vi "abre_help_adq.vi"(1 "nome":string) -> (0 "Erro":bool)   [LabVIEW 2019]
doc: "Este vi abre arquivos pelo Acrobat (.pdf).\nNome PDF - nome do arquivo que deseja abrir. Ele deve estar na subpasta data do mesmo diretório que este vi.\nOk - se false é pq ocorreu algum erro ao procurar o arquivo. Para saber qual erro ocorreu, veja em error out. Caso contrário, o arquivo é aberto."
panel:
  out "appended path":path
  out "error out":errorcluster
  in  "error in (no error)":errorcluster
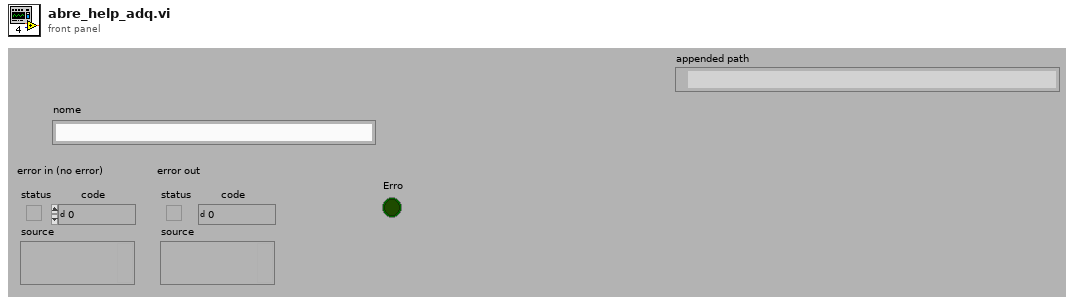
[diagram p1: front panel]
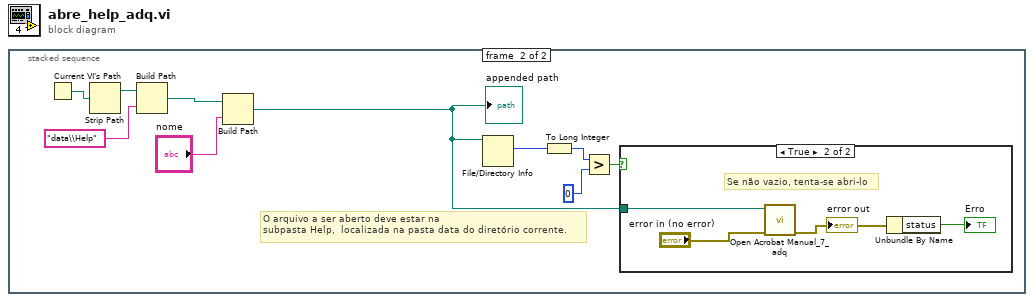
[diagram p0: block diagram]
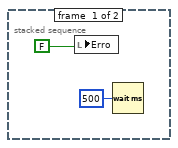
[diagram p2: hidden frame]
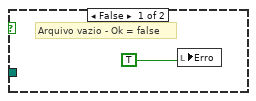
[diagram p3: hidden frame]
diagram:
  n1 = stacked-sequence {
    frame #0 {
      n2 = local write "Erro"(FALSE) -> ()
      n3 = Wait (ms)(milliseconds to wait=u32 500) -> ()  [unwired: 1 out]
    }
    frame #1 {
      # "O arquivo a ser aberto deve estar na \nsubpasta Help,  localizada na pasta data do diretório corrente."
      n4 = Current VI's Path() -> (path=w7:path)
      n5 = Strip Path(path=w7) -> (stripped path=w6:path)  [unwired: 1 out]
      n6 = Build Path(base path=w6, name or relative path="data\\Help") -> (appended path=w4:path)
      n7 = Build Path(base path=w4, name or relative path="nome") -> (appended path=w3:path)
      "appended path" <- w3
      n8 = File/Directory Info(path=w3) -> (size=w8:i64)  [unwired: 1 in, 6 out]
      n9 = To Long Integer(number=w8) -> (32bit integer=w10:i32)
      n10 = Greater?(x=w10, y=0) -> (0:w12:bool)
      n11 = case shown="True" w12 {
        tunnel: w3 -> [_ w17]
        frame False {
          # "Arquivo vazio - Ok = false"
          n12 = local write "Erro"(TRUE) -> ()
        }
        frame True {
          # "Se não vazio, tenta-se abri-lo"
          n13 = call "Open Acrobat Manual_7_adq.vi"("error in (no error)"="error in (no error)", "acrobat document"=w17) -> ("error out"=w15:errorcluster)  [unwired: 5 in]
          "error out" <- w15
          n14 = Unbundle By Name(w15) -> ("status"=→"Erro":bool)
        }
      }
    }
  }
